vi "LeftClick.vi"(6 "Double Click":bool, 7 "Table History ref":refnum<vi>, 8 "error in (no error)":errorcluster, 9 "Table CtlRef In":refnum<vi>, 10 "Cell Position":T1, 11 "Column in":refnum<class "Column.lvclass">) -> (0 "error out":errorcluster, 1 "Table CtlRef Out":refnum<vi>, 2 "Discard?":bool, 3 "Column out":refnum<class "Column.lvclass">, 5 "Button":u16=1)   [LabVIEW 2013, in "Column.lvclass"]
doc: "For a \"standard\" column, let LabVIEW handle by default. Left-click brings up edit, right-click a shortcut menu. This VI is read only w.r.t the column object."
uses:
  Column.lvclass
  <vilib>/Utility/miscctls.llb/LVRowAndColumnTypeDef.ctl
  TypeDefs/TableHistory.ctl
  TypeDefs/TableArray.ctl
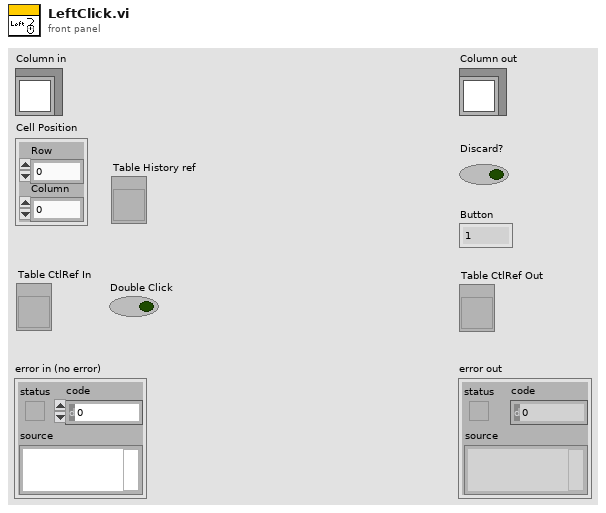
[diagram p1: front panel]
types:
  T1 = typedef "LVRowAndColumnTypeDef.ctl" = cluster{"Row":i32, "Column":i32}
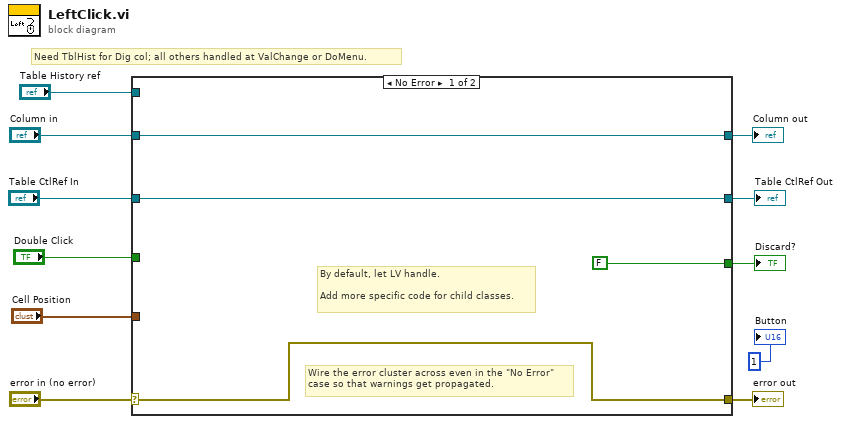
[diagram p0: block diagram]
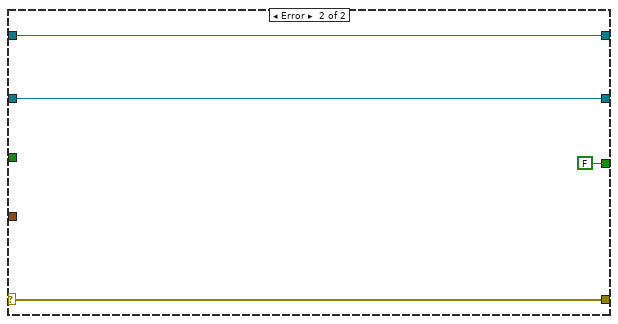
[diagram p2: hidden frame]
diagram:
  # "Need TblHist for Dig col; all others handled at ValChange or DoMenu."
  n1 = case shown="No Error" "error in (no error)" {
    selector: "error in (no error)" -> [w13 w19]
    tunnel: [w13 w19] -> w10
    tunnel: [w15 w18] -> w8
    tunnel: "Column in" -> [w15 w18]
    tunnel: [w12 w17] -> w6
    tunnel: "Table CtlRef In" -> [w12 w17]
    tunnel: "Cell Position" -> [_ _]
    tunnel: "Table History ref" -> [_ _]
    tunnel: "Double Click" -> [_ _]
    tunnel: [FALSE FALSE] -> w1
    frame No Error {
      # "By default, let LV handle.\n\nAdd more specific code for child classes."
      # "Wire the error cluster across even in the \"No Error\"\ncase so that warnings get propagated."
    }
    frame Error {
    }
  }
  "error out" <- w10
  "Column out" <- w8
  "Discard?" <- w1
  "Table CtlRef Out" <- w6
  "Button" <- u16 1 ("Button")
